vi "Read section.vi"(8 "error in (no error)":errorcluster, 11 "Read File Tests in":refnum<class "Read File Tests.lvclass">) -> (0 "error out":errorcluster, 2 "section":string, 3 "Read File Tests out":refnum<class "Read File Tests.lvclass">)   [LabVIEW 2017, in "Read File Tests.lvclass"]
uses:
  Read File Tests.lvclass
  Read File Tests.lvclass/Read File Tests.ctl
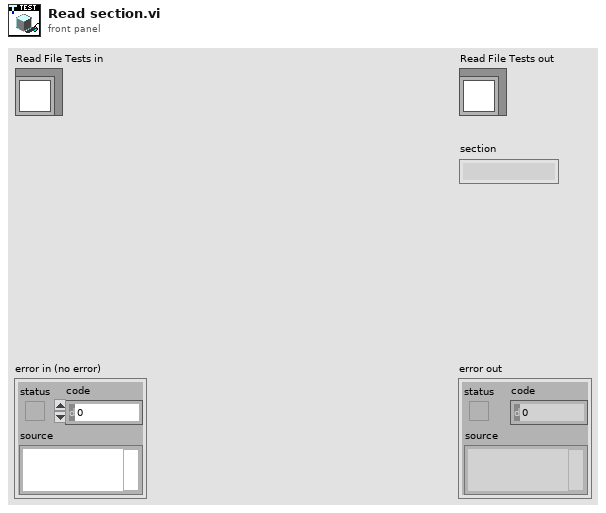
[diagram p1: front panel]
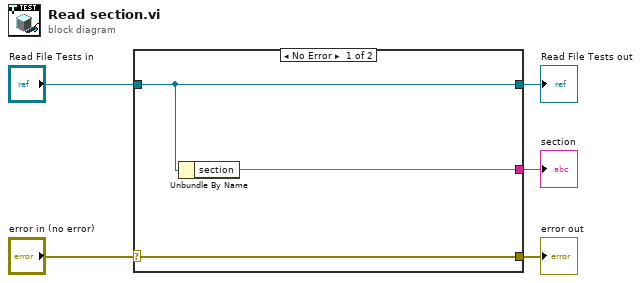
[diagram p0: block diagram]
diagram:
  n1 = case shown="No Error" "error in (no error)" {
    selector: "error in (no error)" -> [w8 w9]
    tunnel: [w8 w9] -> w4
    tunnel: [w7 w10] -> w2
    tunnel: "Read File Tests in" -> [w7 w10]
    tunnel: [w6 _] -> w1
    frame No Error {
      n2 = Unbundle By Name(w7) -> ("section"=w6:string)
    }
    frame Error {
    }
  }
  "error out" <- w4
  "Read File Tests out" <- w2
  "section" <- w1
